vi "W9Q1.vi"() -> ()   [LabVIEW 2021]
uses:
  <vilib>/express/express analysis/Spectral/XNode/ExpressSpectralMeasurementsBlockNode.xnode
  <vilib>/express/express analysis/Spectral/Block/exnSpectralBlock spectral measurements RMS poly.vi
  <vilib>/express/express analysis/Spectral/Block/exnSpectralBlock spectral measurements RMS DDT.vi
panel:
  out "specific":dbl
  out "RMS":dbl
  out "THD":dbl
  out "Peak":dbl
  out "Waveform Graph 2":dynamicdata(graph)
  out "Waveform Graph":dynamicdata(graph)
  in  "stop":bool
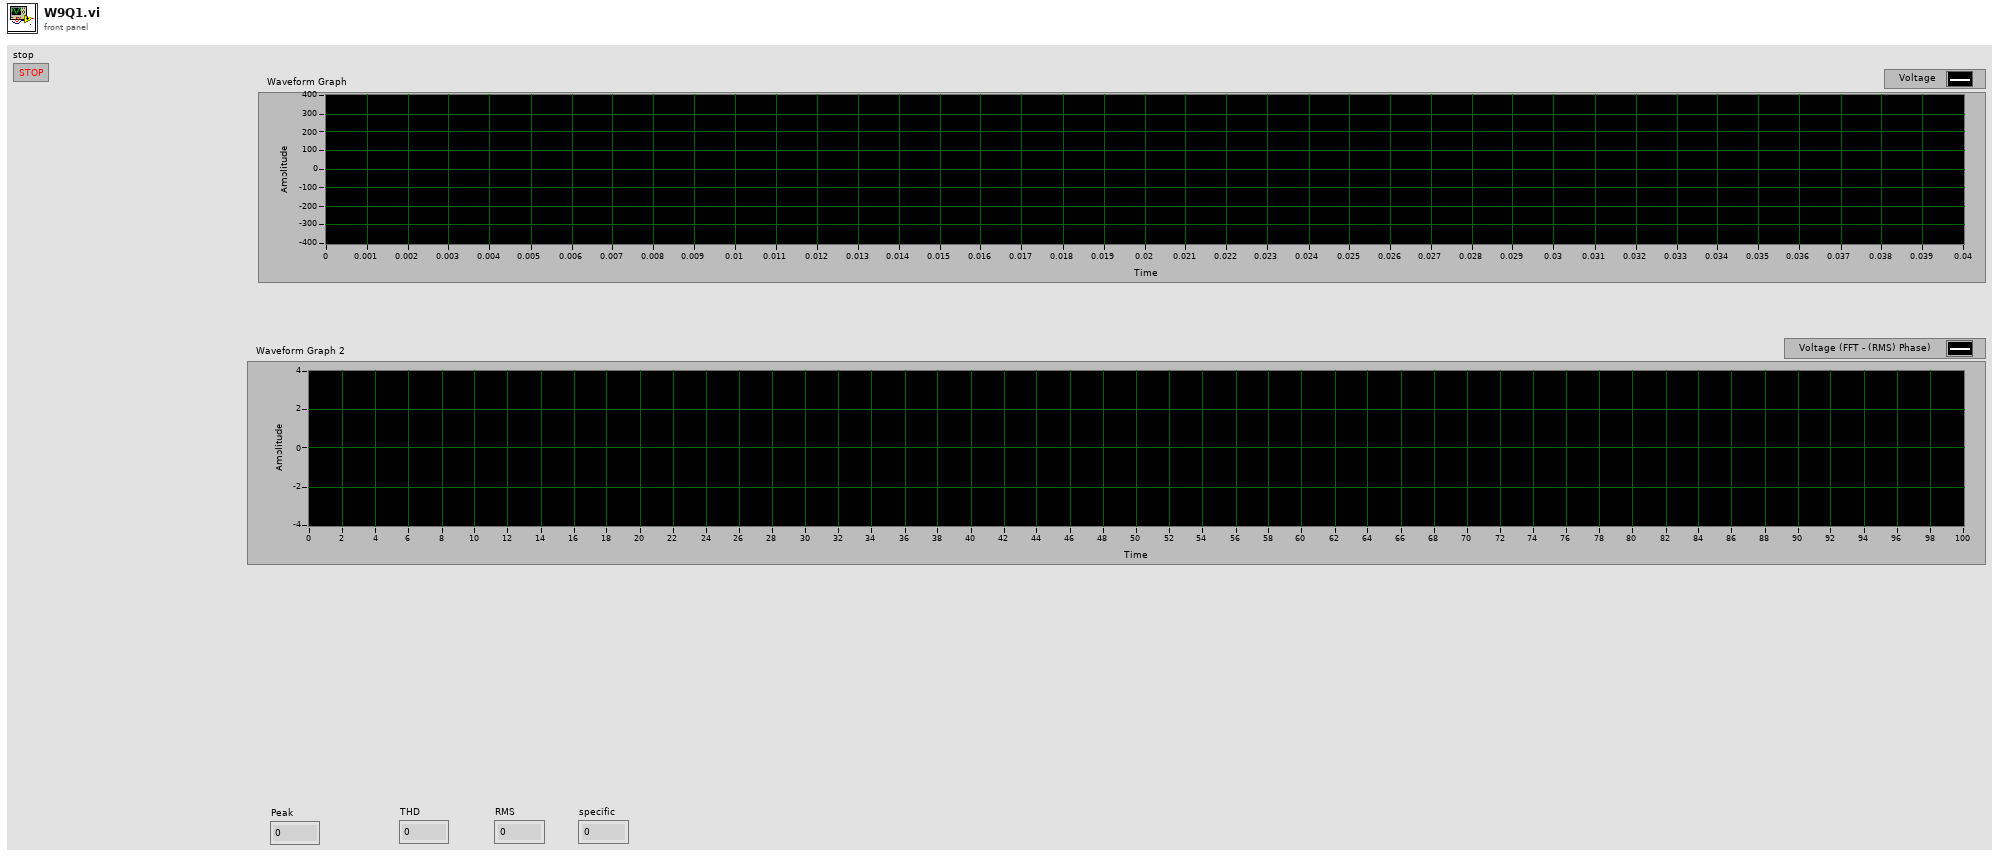
[diagram p1: front panel]
types:
  T1 = cluster{"averaging mode":u16, "weighting mode":u16, "number of averages":u32}
  T2 = cluster{"dB On (F)":bool, "unwrap phase (F)":bool, "convert to degree (F)":bool}
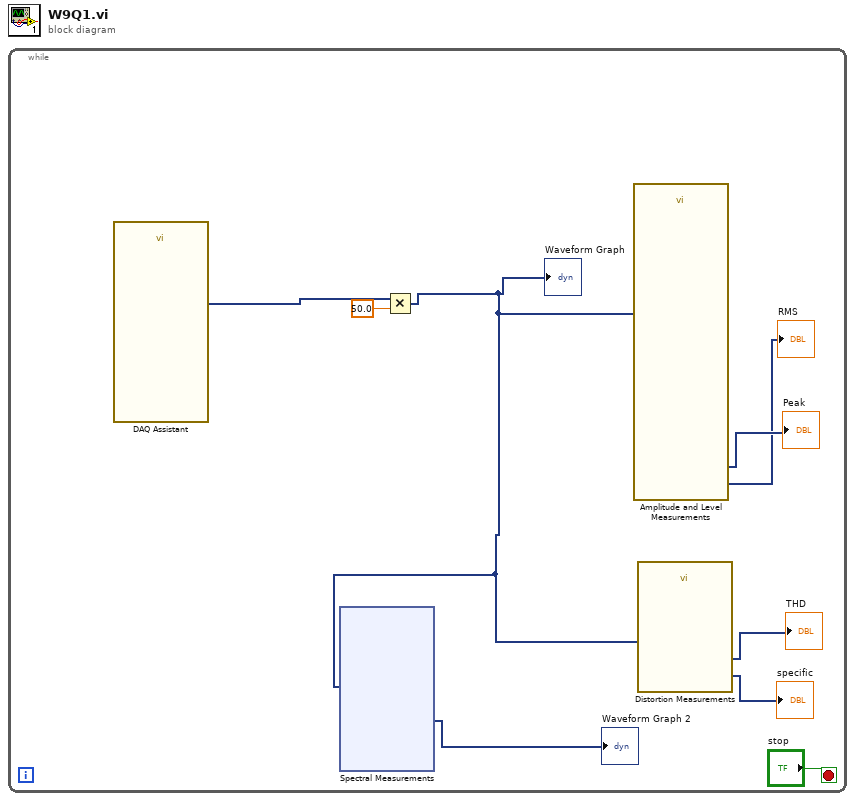
[diagram p0: block diagram]
diagram:
  n1 = while {
    stop <- "stop" stop-if-true
    n2 = call "DAQ Assistant"() -> ("data"=w8:dynamicdata)  [unwired: 16 in, 3 out]
    n3 = Multiply(x=w8, y=50.0) -> (x*y=w6:dynamicdata)
    "Waveform Graph" <- w6
    n4 = xnode "Spectral Measurements"("Signals"=w6) -> ("Phase"=→"Waveform Graph 2":dynamicdata)  [unwired: 1 in, 2 out]
    n5 = call "Amplitude and Level Measurements"("Signals"=w6) -> ("RMS"=→"RMS":dynamicdata, "Positive Peak"=→"Peak":dynamicdata)  [unwired: 7 in, 6 out]
    n6 = call "Distortion Measurements"("Signals"=w6) -> ("Specific Harmonic"=→"specific":dynamicdata, "THD"=→"THD":dynamicdata)  [unwired: 8 in, 1 out]
  }
